vi "Main.vi"() -> ()   [LabVIEW 2020]
uses:
  States.ctl
  <vilib>/MakerHub/LINX/Public/Utilities/Open Serial.vi
  <vilib>/MakerHub/LINX/Public/Sensors/Motion/Servo/Servo Open One Channel.vi
  <vilib>/MakerHub/LINX/Public/Sensors/Motion/Servo/Servo Close One Channel.vi
  <vilib>/MakerHub/LINX/LMH-LINX.lvlib
  <vilib>/MakerHub/LINX/Public/Sensors/Motion/Servo/Servo.lvlib
panel:
  out "door":u16(ring)
  in  "Serial Port":refnum<visa-resource-name>="N/A"
  in  "Buzzer":u8=5
  in  "Servo":u8=6
  in  "stop":bool
  in  "2":bool
  in  "3":bool
  in  "4":bool
  in  "5":bool
  in  "6":bool
  in  "7":bool
  in  "8":bool
  in  "9":bool
  in  "0":bool
  in  "1":bool
  out "String":string
  # "Controls"
  # "Password : 3333"
  # "Wait 5 sec before start"
  # "Serial Port"
  # "Servo"
  # "Buzzer"
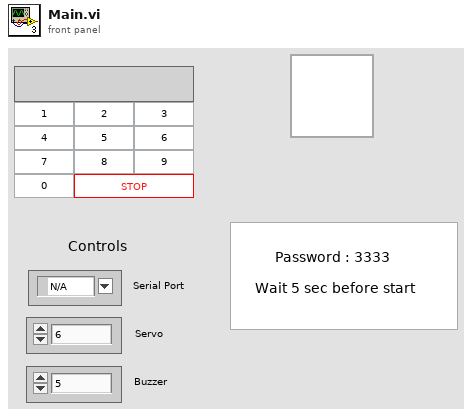
[diagram p1: front panel]
types:
  T1 = typedef "States.ctl" = enum16{"Main", "Check", "Correct", "Wrong", "Too Wrong"}
  T2 = typedef "LMH-LINX.lvlib/LINX Ref.ctl" = cluster{"IO":T3, "Interface":T4, "LINX Device Config":T5}
  T3 = typedef "LMH-LINX.lvlib/Platform.ctl" = enum16{"Remote", "Local"}
  T4 = typedef "LMH-LINX.lvlib/Interface.ctl" = enum16{"Serial", "TCP"}
  T5 = typedef "LMH-LINX.lvlib/Device.lvlib/LINX Device Config.ctl" = cluster{"Interface":T4, "COM Port":refnum<visa-resource-name>, "TCP Configuration":T6, "Device Family":u8, "Device ID":u8, "Device Name":string, "TCP Ref":refnum<k5>, "Channels":T7}
  T6 = typedef "LMH-LINX.lvlib/Device.lvlib/TCP Config.ctl" = cluster{"IP Address":string, "Port":u16}
  T7 = typedef "LMH-LINX.lvlib/Channels.ctl" = cluster{"DI":u8[], "DO":u8[], "AI":u8[], "AO":u8[], "PWM":u8[], "QE":u8[], "UART":u8[], "I2C 2":u8[], "SPI":u8[], "CAN":u8[], "Servo":u8[], "AI Ref (V)":dbl, "AI Resolution (Bits)":u8, "AO Ref (V)":dbl, "AO Resolution (Bits)":u8}
  T8 = enum8{"Enabled", "Disabled", "Disabled and Grayed Out"}
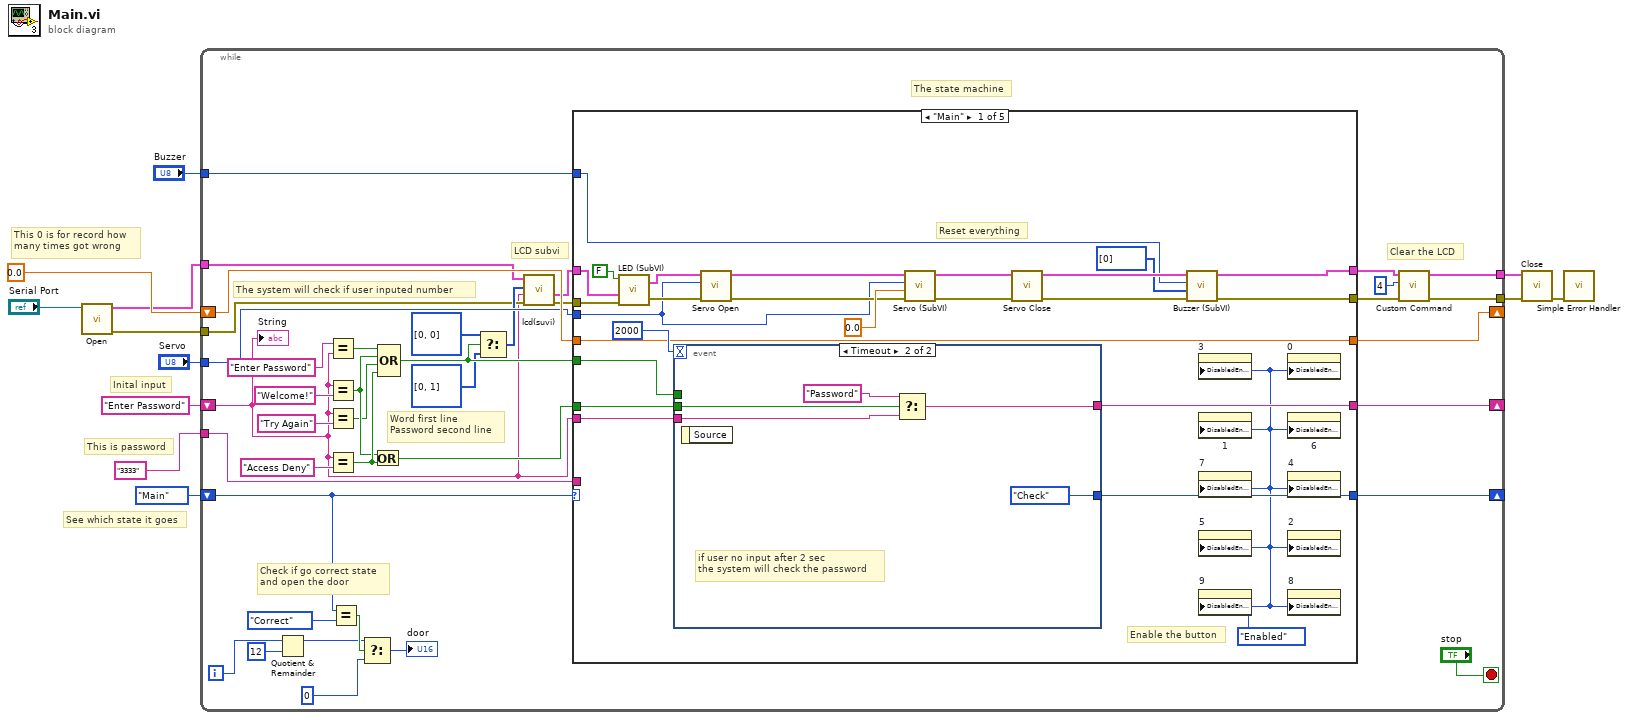
[diagram p0: block diagram]
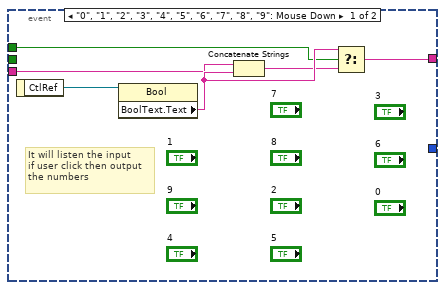
[diagram p2: hidden frame]
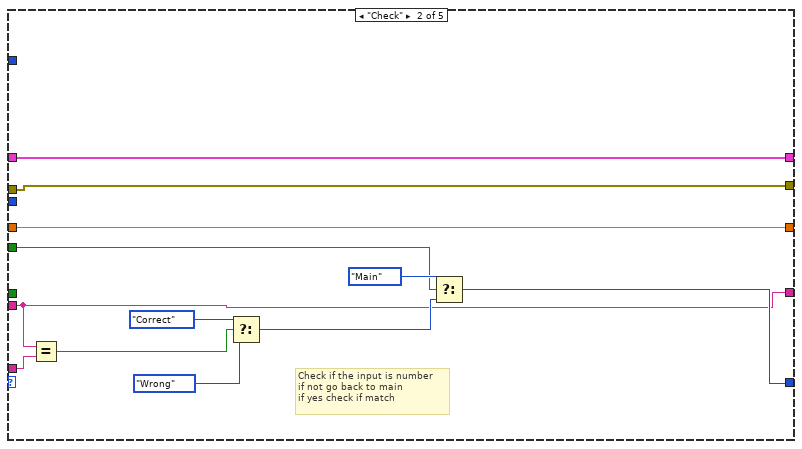
[diagram p3: hidden frame]
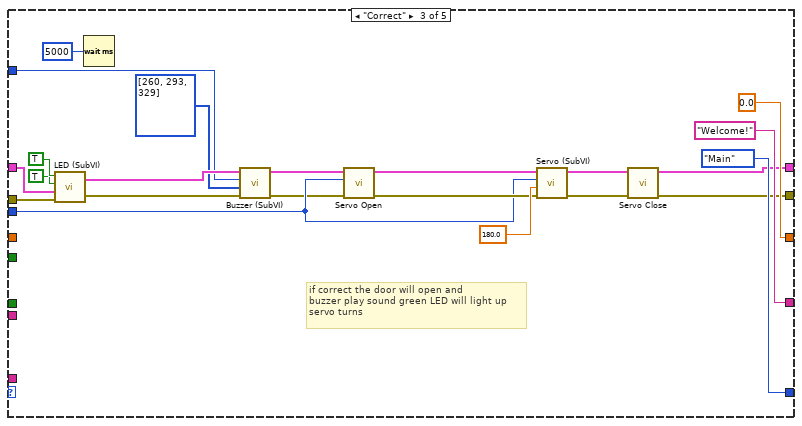
[diagram p4: hidden frame]
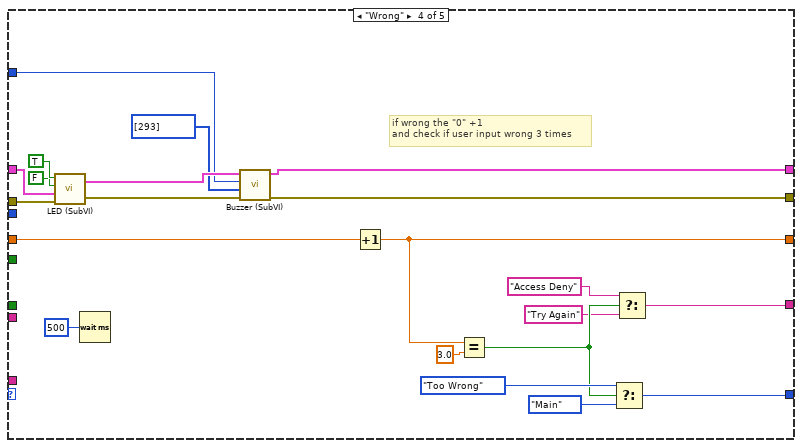
[diagram p5: hidden frame]
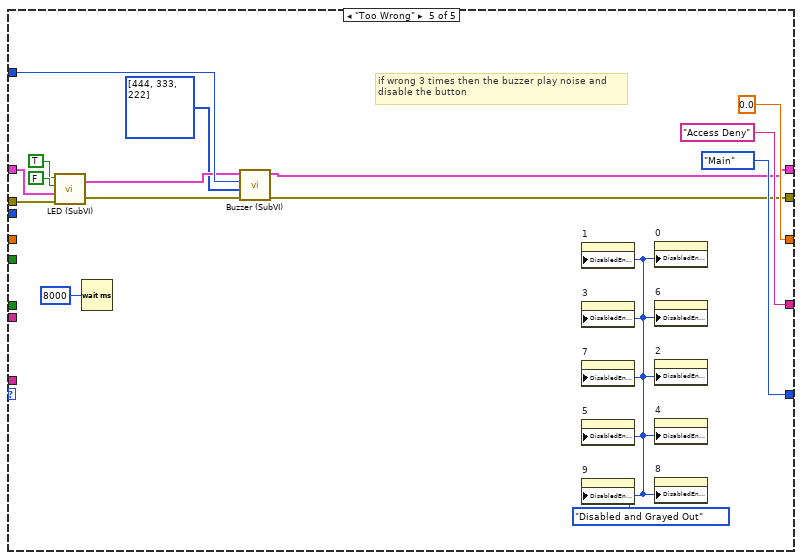
[diagram p6: hidden frame]
diagram:
  # "This 0 is for record how \nmany times got wrong"
  # "Inital input"
  # "See which state it goes"
  # "This is password"
  n1 = call-poly <vilib>:"Open.vi"("Serial Port"="Serial Port") -> ("Error Out"=w4:errorcluster, "LINX Resource"=w5:T2)  [unwired: 8 in, 1 out]
  n2 = while {
    shift-right: [w51] -> _
    shift-left: States."Main" -> [w21]
    shift-right: [w47] -> _
    shift-left: "Enter Password" -> [w13]
    shift-right: [w48] -> _
    shift-left: 0.0 -> [w49]
    tunnel: w5 -> [w29]
    tunnel: w4 -> [w28]
    tunnel: "Servo" -> [w46]
    tunnel: "3333" -> [w45]
    tunnel: "Buzzer" -> [w44]
    tunnel: [w25] -> w2
    tunnel: [w22] -> w1
    i -> [w16]
    stop <- "stop" stop-if-true
    # "Clear the LCD"
    # "Word first line\nPassword second line"
    # "The system will check if user inputed number"
    # "LCD subvi"
    # "The state machine"
    # "Check if go correct state\nand open the door"
    n3 = Quotient & Remainder(x=w16, y=12) -> (x-y*floor(x/y)=w17:i32)  [unwired: 1 out]
    n4 = Equal?(x="Enter Password", y=w13) -> (x = y?=w41:bool)
    n5 = Equal?(x=w13, y="Welcome!") -> (x = y?=w42:bool)
    n6 = Equal?(x=w13, y="Try Again") -> (x = y?=w40:bool)
    n7 = Equal?(x=w13, y="Access Deny") -> (x = y?=w43:bool)
    n8 = Equal?(x=w21, y=States."Correct") -> (x = y?=w18:bool)
    n9 = Select(t=w17, s=w18, f=0 ("y")) -> (s? t:f=→"door":i32)
    n10 = Or(x=w42, y=w43) -> (x .or. y?=w35:bool)
    n11 = Compound Arithmetic op=OR(w41, w42, w40, w43) -> (w33:bool)
    n12 = Select(t=u8[] [0, 0] ("location"), s=w33, f=u8[] [0, 1] ("location")) -> (s? t:f=w30:u8[])
    n13 = call "lcd(suvi).vi"("error in (no error)"=w28, "String"=w13, "location"=w30, "LINX Resource in"=w29) -> ("error out"=w23:errorcluster, "LINX Resource"=w24:T2)  [unwired: 4 in, 2 out]
    n14 = case shown="\"Main\"" w21 {
      tunnel: [w76 w93 States."Main" w138 States."Main"] -> w51
      tunnel: w13 -> [w75 w92 _ _ _]
      tunnel: w49 -> [w72 w97 _ w142 _]
      tunnel: [w72 w97 0.0 w141 0.0] -> w48
      tunnel: [w74 w92 "Welcome!" w133 "Access Deny"] -> w47
      tunnel: w24 -> [w65 w91 w118 w132 w151]
      tunnel: w23 -> [w64 w90 w117 w131 w150]
      tunnel: [w55 w91 w109 w123 w144] -> w27
      tunnel: [w54 w90 w108 w122 w143] -> w26
      tunnel: w46 -> [w61 _ w107 _ _]
      tunnel: w45 -> [_ w89 _ _ _]
      tunnel: w44 -> [w56 _ w103 w124 w148]
      tunnel: w35 -> [w53 _ _ _ _]
      tunnel: w33 -> [w52 w88 _ _ _]
      frame "Main" {
        w60 = T8."Enabled" ("Disabled")
        # "Reset everything"
        # "Enable the button"
        n15 = call "LED (SubVI).vi"("error in (no error)"=w64, "LINX Resource in"=w65, "On/OFF"=FALSE) -> ("error out"=w62:errorcluster, "LINX Resource out"=w63:T2)  [unwired: 1 in]
        n16 = event shown="[1] Timeout" {
          selector: _ -> [_ _]
          dyn-events: _ -> [_ _]
          timeout: 2000 -> [_ _]
          tunnel: [_ States."Check"] -> w76
          tunnel: w75 -> [w78 w84]
          tunnel: [w80 w85] -> w74
          tunnel: w52 -> [w77 _]
          tunnel: w53 -> [_ w83]
          event "0", "1", "2", "3", "4", "5", "6", "7", "8", "9": Mouse Down {
            # "It will listen the input\nif user click then output\nthe numbers"
            n17 = event-data() -> ("CtlRef"=w82:refnum<vi>)  [unwired: 1 in]
            n18 = property class="Bool"(reference=w82) -> ("BoolText.Text"=w81:string)  [unwired: 1 in, 2 out]
            n19 = Concatenate Strings(w78, w81) -> (w79:string)
            n20 = Select(t=w81, s=w77, f=w79) -> (s? t:f=w80:string)
          }
          event Timeout {
            # "if user no input after 2 sec\nthe system will check the password"
            n21 = event-data() -> ()  [unwired: 1 in, 1 out]
            n22 = Select(t="Password", s=w83, f=w84) -> (s? t:f=w85:string)
          }
        }
        n23 = call-poly <vilib>:"Servo Open.vi"("Error In"=w62, "Servo Channel"=w61, "LINX Resource"=w63) -> ("Error Out"=w68:errorcluster, "LINX Resource"=w69:T2)  [unwired: 7 in]
        n24 = call "Servo (SubVI).vi"("error in (no error)"=w68, "Position in"=0.0, "Servo Channel"=w61, "LINX Resource in"=w69) -> ("error out"=w66:errorcluster, "LINX Resource out"=w67:T2)  [unwired: 5 in, 1 out]
        n25 = call-poly <vilib>:"Servo Close.vi"("Error In"=w66, "LINX Resource"=w67) -> ("Error Out"=w58:errorcluster, "LINX Resource"=w59:T2)  [unwired: 8 in]
        n26 = call "Buzzer (SubVI).vi"("error in (no error)"=w58, "Array"=i32[] [0], "Digital Pin"=w56, "LINX Resource in"=w59) -> ("error out"=w54:errorcluster, "LINX Resource out"=w55:T2)  [unwired: 6 in]
        n27 = property on="3" class="Bool"("DisabledEnum"=w60) -> ()  [unwired: 2 in, 2 out]
        n28 = property on="1" class="Bool"("DisabledEnum"=w60) -> ()  [unwired: 2 in, 2 out]
        n29 = property on="7" class="Bool"("DisabledEnum"=w60) -> ()  [unwired: 2 in, 2 out]
        n30 = property on="5" class="Bool"("DisabledEnum"=w60) -> ()  [unwired: 2 in, 2 out]
        n31 = property on="9" class="Bool"("DisabledEnum"=w60) -> ()  [unwired: 2 in, 2 out]
        n32 = property on="0" class="Bool"("DisabledEnum"=w60) -> ()  [unwired: 2 in, 2 out]
        n33 = property on="6" class="Bool"("DisabledEnum"=w60) -> ()  [unwired: 2 in, 2 out]
        n34 = property on="4" class="Bool"("DisabledEnum"=w60) -> ()  [unwired: 2 in, 2 out]
        n35 = property on="2" class="Bool"("DisabledEnum"=w60) -> ()  [unwired: 2 in, 2 out]
        n36 = property on="8" class="Bool"("DisabledEnum"=w60) -> ()  [unwired: 2 in, 2 out]
      }
      frame "Check" {
        # "Check if the input is number\nif not go back to main\nif yes check if match"
        n37 = Equal?(x=w92, y=w89) -> (x = y?=w96:bool)
        n38 = Select(t=States."Correct", s=w96, f=States."Wrong") -> (s? t:f=w94:T1)
        n39 = Select(t=States."Main", s=w88, f=w94) -> (s? t:f=w93:T1)
      }
      frame "Correct" {
        # "if correct the door will open and \nbuzzer play sound green LED will light up\nservo turns"
        n40 = call "LED (SubVI).vi"("error in (no error)"=w117, "LINX Resource in"=w118, "Blue / Red"=TRUE ("Green/Red"), "On/OFF"=TRUE) -> ("error out"=w104:errorcluster, "LINX Resource out"=w105:T2)
        n41 = Wait (ms)(milliseconds to wait=u32 5000 ("millisecond multiple")) -> ()  [unwired: 1 out]
        n42 = call "Buzzer (SubVI).vi"("error in (no error)"=w104, "Array"=i32[] [260, 293, 329], "Digital Pin"=w103, "LINX Resource in"=w105) -> ("error out"=w100:errorcluster, "LINX Resource out"=w101:T2)  [unwired: 6 in]
        n43 = call-poly <vilib>:"Servo Open.vi"("Error In"=w100, "Servo Channel"=w107, "LINX Resource"=w101) -> ("Error Out"=w112:errorcluster, "LINX Resource"=w113:T2)  [unwired: 7 in]
        n44 = call "Servo (SubVI).vi"("error in (no error)"=w112, "Position in"=180.0, "Servo Channel"=w107, "LINX Resource in"=w113) -> ("error out"=w110:errorcluster, "LINX Resource out"=w111:T2)  [unwired: 5 in, 1 out]
        n45 = call-poly <vilib>:"Servo Close.vi"("Error In"=w110, "LINX Resource"=w111) -> ("Error Out"=w108:errorcluster, "LINX Resource"=w109:T2)  [unwired: 8 in]
      }
      frame "Wrong" {
        # "if wrong the \"0\" +1 \nand check if user input wrong 3 times"
        n46 = call "LED (SubVI).vi"("error in (no error)"=w131, "LINX Resource in"=w132, "Blue / Red"=FALSE ("Green/Red"), "On/OFF"=TRUE) -> ("error out"=w126:errorcluster, "LINX Resource out"=w127:T2)
        n47 = Wait (ms)(milliseconds to wait=u32 500) -> ()  [unwired: 1 out]
        n48 = call "Buzzer (SubVI).vi"("error in (no error)"=w126, "Array"=i32[] [293], "Digital Pin"=w124, "LINX Resource in"=w127) -> ("error out"=w122:errorcluster, "LINX Resource out"=w123:T2)  [unwired: 6 in]
        n49 = Increment(x=w142) -> (x+1=w141:dbl)
        n50 = Equal?(x=w141, y=3.0) -> (x = y?=w136:bool)
        n51 = Select(t=States."Too Wrong", s=w136, f=States."Main") -> (s? t:f=w138:T1)
        n52 = Select(t="Access Deny", s=w136, f="Try Again") -> (s? t:f=w133:string)
      }
      frame "Too Wrong" {
        w154 = T8."Disabled and Grayed Out" ("Disabled")
        # "if wrong 3 times then the buzzer play noise and\ndisable the button"
        n53 = call "LED (SubVI).vi"("error in (no error)"=w150, "LINX Resource in"=w151, "Blue / Red"=FALSE ("Green/Red"), "On/OFF"=TRUE) -> ("error out"=w146:errorcluster, "LINX Resource out"=w147:T2)
        n54 = Wait (ms)(milliseconds to wait=u32 8000 ("millisecond multiple")) -> ()  [unwired: 1 out]
        n55 = call "Buzzer (SubVI).vi"("error in (no error)"=w146, "Array"=i32[] [444, 333, 222], "Digital Pin"=w148, "LINX Resource in"=w147) -> ("error out"=w143:errorcluster, "LINX Resource out"=w144:T2)  [unwired: 6 in]
        n56 = property on="1" class="Bool"("DisabledEnum"=w154) -> ()  [unwired: 2 in, 2 out]
        n57 = property on="3" class="Bool"("DisabledEnum"=w154) -> ()  [unwired: 2 in, 2 out]
        n58 = property on="7" class="Bool"("DisabledEnum"=w154) -> ()  [unwired: 2 in, 2 out]
        n59 = property on="5" class="Bool"("DisabledEnum"=w154) -> ()  [unwired: 2 in, 2 out]
        n60 = property on="9" class="Bool"("DisabledEnum"=w154) -> ()  [unwired: 2 in, 2 out]
        n61 = property on="0" class="Bool"("DisabledEnum"=w154) -> ()  [unwired: 2 in, 2 out]
        n62 = property on="6" class="Bool"("DisabledEnum"=w154) -> ()  [unwired: 2 in, 2 out]
        n63 = property on="2" class="Bool"("DisabledEnum"=w154) -> ()  [unwired: 2 in, 2 out]
        n64 = property on="4" class="Bool"("DisabledEnum"=w154) -> ()  [unwired: 2 in, 2 out]
        n65 = property on="8" class="Bool"("DisabledEnum"=w154) -> ()  [unwired: 2 in, 2 out]
      }
    }
    n66 = call <vilib>:"Custom Command.vi"("Error In"=w26, "Custom Command Number"=u16 4, "LINX Resource"=w27) -> ("Error Out"=w22:errorcluster, "LINX Resource"=w25:T2)  [unwired: 5 in, 2 out]
    "String" <- w13
  }
  n67 = call <vilib>:"Close.vi"("Error In"=w1, "LINX Resource"=w2) -> ("Error Out"=w9:errorcluster)  [unwired: 9 in]
  n68 = call <vilib>:"Simple Error Handler.vi"("error in (no error)"=w9) -> ()  [unwired: 4 in, 5 out]
